vi "GV_ToolbarDiskType.vi"(7 "Layer":i32, 8 "Hor-pos":i32, 11 "Pict in":picture) -> (0 "x":i16, 1 "y":i16, 3 "Pict out":picture)   [LabVIEW 2020, in "Sgraph_lib_V1.lvlib" / "Gviewer.lvclass"]
doc: "Andre Koelewijn, 20 June 2021\n\nDraw the Memory or Disk icon & memory Layer into the toolbar"
uses:
  Gviewer.lvclass
  <vilib>/picture/picture.llb/imagedata.ctl
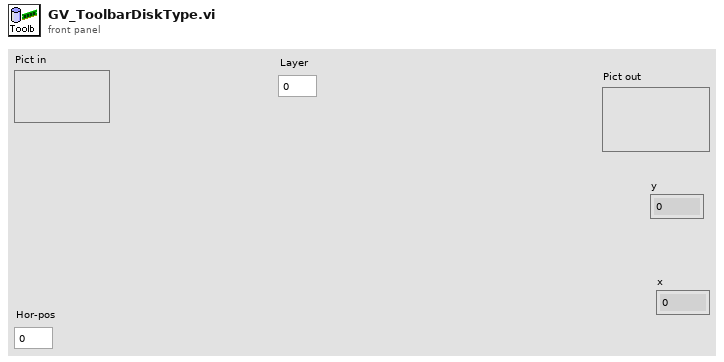
[diagram p1: front panel]
types:
  T1 = cluster{"horizontal":enum16{"left", "center", "right"}, "vertical":enum16{"top", "center", "bottom"}}
  T2 = typedef "imagedata.ctl" = cluster{"image type":i32, "image depth":i32, "image":u8[], "mask":u8[], "colors":u32[], "Rectangle":cluster{"left":i16, "top":i16, "right":i16, "bottom":i16}}
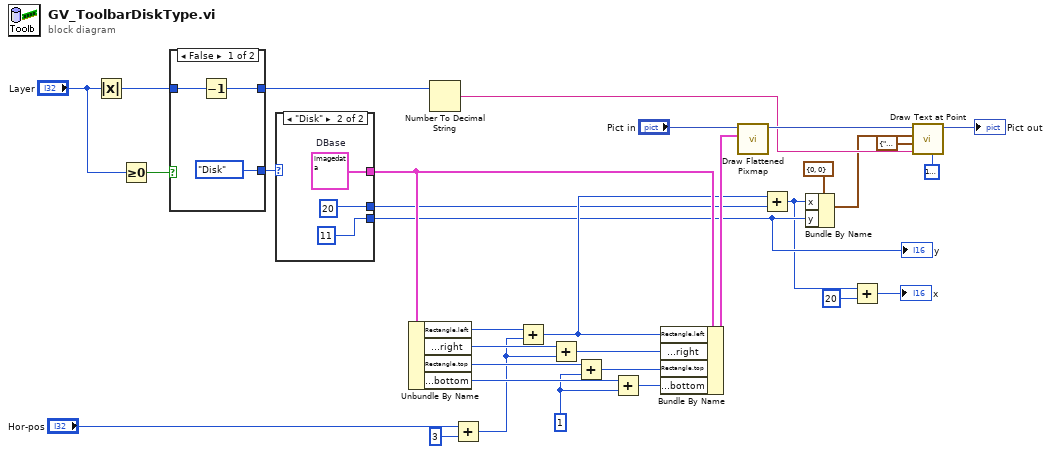
[diagram p0: block diagram]
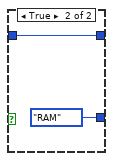
[diagram p2: hidden frame]
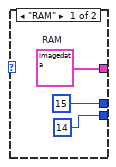
[diagram p3: hidden frame]
diagram:
  w24 = 1
  n1 = Absolute Value(x="Layer") -> (abs(x)=w6:i32)
  n2 = Greater Or Equal To 0?(x="Layer") -> (x >= 0?=w17:bool)
  n3 = case shown="False" w17 {
    tunnel: [enum16{"RAM", "Disk"}."Disk" ("MemoryType") enum16{"RAM", "Disk"}."RAM" ("MemoryType")] -> w18
    tunnel: w6 -> [w34 w36]
    tunnel: [w33 w36] -> w5
    frame False {
      n4 = Decrement(x=w34) -> (x-1=w33:i32)
    }
    frame True {
    }
  }
  n5 = case shown="\"Disk\"" w18 {
    tunnel: [w40 w43] -> w30
    tunnel: [i16 14 ("y") i16 11 ("y")] -> w8
    tunnel: [15 ("y") 20 ("y")] -> w7
    frame "RAM" {
      w40 = T2 {"image type"=0, "image depth"=32, "image"=array[3360 elements], "mask"=[0, 0, 0, 0, 4, 8, 32, 128, 14, 28, 113, 192, 14, 28, 113, 192, 14, 28, 113, 192, 63, 255, 255, 240, 127, 255, 255, 248, 127, 255, 255, 248, 127, 255, 255, 248, 127, 255, 255, 248, 127, 255, 255, 248, 127, 255, 255, 248, 127, 255, 255, 248, 127, 255, 255, 248, 127, 255, 255, 248, 127, 255, 255, 248, 127, 255, 255, 248, 127, 255, 255, 248, 127, 255, 255, 248, 127, 255, 255, 248, 127, 255, 255, 248, 127, 255, 255, 248, 63, 255, 255, 240, 14, 56, 227, 128, 14, 56, 227, 128, 14, 56, 227, 128, 4, 16, 65, 0, 0, 0, 0, 0], "colors"=[], "Rectangle"={"left"=0, "top"=0, "right"=30, "bottom"=28}}  # RAM
    }
    frame "Disk" {
      w43 = T2 {"image type"=0, "image depth"=32, "image"=array[3472 elements], "mask"=[0, 0, 0, 0, 15, 255, 255, 192, 16, 0, 0, 48, 32, 0, 0, 16, 33, 240, 0, 8, 35, 248, 0, 8, 39, 252, 0, 8, 39, 252, 0, 8, 39, 252, 0, 8, 39, 252, 0, 8, 39, 252, 0, 8, 39, 252, 0, 8, 39, 252, 0, 8, 39, 252, 0, 8, 39, 252, 0, 8, 35, 248, 0, 8, 33, 240, 0, 8, 32, 0, 0, 16, 24, 0, 0, 48, 7, 255, 255, 192, 0, 1, 0, 0, 0, 1, 0, 0, 0, 3, 128, 0, 0, 4, 64, 0, 63, 252, 127, 248, 0, 4, 64, 0, 0, 3, 128, 0, 0, 0, 0, 0], "colors"=[], "Rectangle"={"left"=0, "top"=0, "right"=31, "bottom"=28}}  # DBase
    }
  }
  "y" <- w8
  n6 = Unbundle By Name(w30) -> ("Rectangle.left"=w32:i16, "Rectangle.right"=w31:i16, "Rectangle.top"=w27:i16, "Rectangle.bottom"=w25:i16)
  n7 = Number To Decimal String(number=w5) -> (decimal integer string=w13:string)  [unwired: 1 in]
  n8 = Add(x="Hor-pos", y=3) -> (x+y=w19:i32)
  n9 = Add(x=w32, y=w19) -> (x+y=w9:i32)
  n10 = Add(x=w31, y=w19) -> (x+y=w28:i32)
  n11 = Add(x=w27, y=w24) -> (x+y=w26:i32)
  n12 = Add(x=w25, y=w24) -> (x+y=w23:i32)
  n13 = Bundle By Name(cluster=w30, "Rectangle.left"=w9, "Rectangle.right"=w28, "Rectangle.top"=w26, "Rectangle.bottom"=w23) -> (w29:T2)
  n14 = call <vilib>:"Draw Flattened Pixmap.vi"("image data"=w29, "picture"="Pict in") -> ("new picture"=w16:picture)  [unwired: 7 in]
  n15 = Add(x=w9, y=w7) -> (x+y=w4:i32)
  n16 = Bundle By Name(cluster=cluster{"x":i16, "y":i16} {"x"=0, "y"=0} ("origin"), "x"=w4, "y"=w8) -> (w10:cluster{"x":i16, "y":i16})
  n17 = Add(x=w4, y=20) -> (x+y=→"x":i32)
  n18 = call <vilib>:"Draw Text at Point.vi"("BG color(transparent)"=u32 16777216, "text"=w13, "alignment(left, top)"=T1 {"horizontal"=enum."center", "vertical"=enum."center"}, "origin"=w10, "picture"=w16) -> ("new picture"=→"Pict out":picture)  [unwired: 5 in, 1 out]
